vi "Do.vi"(8 "error in":errorcluster, 10 "Actor in":refnum<class "Actor.lvclass">, 11 "Send Command MSG":refnum<class "Send Command MSG.lvclass">) -> (0 "error out":errorcluster, 2 "Actor out":refnum<class "Actor.lvclass">)   [LabVIEW 2017, in "Send Command MSG.lvclass"]
doc: "(<B>Filename</B>: Actor Framework.lvlib:Message.lvclass:Do.vi)\n\nDefines what a message does when it is received by an actor. Generally, a message instructs an actor to invoke one of its methods. By default, this method does nothing. A child class must override it to define behavior. Create a child class by using the Actor Framework Message Maker dialog box."
uses:
  Send Command MSG.lvclass
  <vilib>/ActorFramework/Actor/Actor.lvclass
  <vilib>/MSR Consulting, LLC/General Reuse/Instrument/Actor/Instrument Actor.lvclass
  C:/Program Files (x86)/National Instruments/LabVIEW 2017/vi.lib/ActorFramework/Actor/Actor.lvclass
  <vilib>/MSR Consulting, LLC/General Reuse/Instrument/Actor/Instrument Actor.lvclass/Instrument Actor.ctl
  <vilib>/MSR Consulting, LLC/General Reuse/Instrument/Instrument.lvclass/Instrument.ctl
  Send Command MSG.lvclass/Send Command MSG.ctl
  <vilib>/MSR Consulting, LLC/General Reuse/Instrument/Actor/Read Instr.vi
  <vilib>/MSR Consulting, LLC/General Reuse/Instrument/Read CMD.vi
  <vilib>/MSR Consulting, LLC/General Reuse/Instrument/Instrument.lvclass
  <vilib>/MSR Consulting, LLC/General Reuse/Command/Command.lvclass
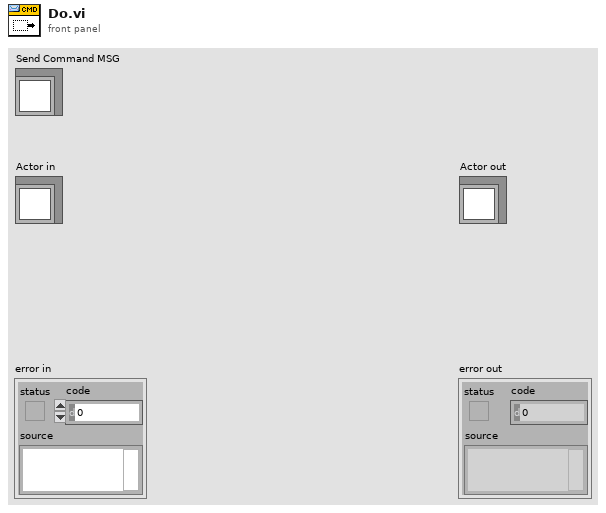
[diagram p1: front panel]
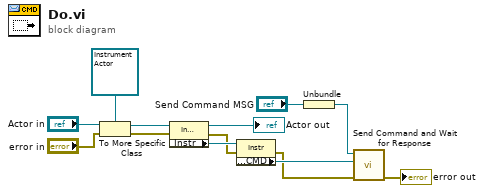
[diagram p0: block diagram]
diagram:
  n1 = To More Specific Class(target class=refnum<class "Instrument Actor.lvclass"> refnum ("Instrument Actor"), reference="Actor in", error in="error in") -> (specific class reference=w10:refnum<class "Instrument Actor.lvclass">, error out=w6:errorcluster)
  n2 = property class="Instrument Actor"(reference=w10, error in=w6) -> (reference out=→"Actor out":refnum<class "Instrument Actor.lvclass">, error out=w5:errorcluster, "Instr"=w8:refnum<class "Instrument.lvclass">)
  n3 = property class="Instr"(reference=w8, error in=w5) -> (error out=w2:errorcluster, "Accessors:CMD"=w3:refnum<queue>)  [unwired: 1 out]
  n4 = Unbundle("Send Command MSG") -> (w4:refnum<class "Command.lvclass">)
  n5 = call <vilib>:"Send Command and Wait for Response.vi"("error in"=w2, "cmd queue"=w3, "CMD in"=w4) -> ("error out"=→"error out":errorcluster)  [unwired: 6 in, 2 out]
